vi "DevTests_TestEvent.vi"() -> ()   [LabVIEW 2024]
uses:
  SDL3/Video/WindowFlags--ring.ctl
  SDL3/Pixels/PixelFormat--enum.ctl
  SDL3/Render/TextureAccess-enum.ctl
  SDL3/Error/GetError-UiThread.vi
  SDL3/Pixels/PixelFormatEnumToU32.vi
  <vilib>/Utility/error.llb/Error Cluster From Error Code.vi
  SDL3/Render/Render.lvlib
  SDL3/Init/Init.lvlib
  SDL3/Video/Video.lvlib
  SDL3/Pixels/Pixels.lvlib
  SDL3/Events/Events.lvlib
panel:
  in  "stop":bool
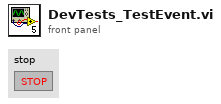
[diagram p1: front panel]
types:
  T1 = typedef "SDL3.lvlib/Render.lvlib/TextureAccess-enum.ctl" = enum32{"SDL_TEXTUREACCESS_STATIC", "SDL_TEXTUREACCESS_STREAMING", "SDL_TEXTUREACCESS_TARGET"}
  T2 = typedef "SDL3.lvlib/Pixels.lvlib/PixelFormat--enum.ctl" = enum32{"SDL_PIXELFORMAT_UNKNOWN", "SDL_PIXELFORMAT_INDEX1LSB", "SDL_PIXELFORMAT_INDEX1MSB", "SDL_PIXELFORMAT_INDEX2LSB", "SDL_PIXELFORMAT_INDEX2MSB", "SDL_PIXELFORMAT_INDEX4LSB", "SDL_PIXELFORMAT_INDEX4MSB", "SDL_PIXELFORMAT_INDEX8", "SDL_PIXELFORMAT_RGB332", "SDL_PIXELFORMAT_XRGB4444", "SDL_PIXELFORMAT_XBGR4444", "SDL_PIXELFORMAT_XRGB1555", "SDL_PIXELFORMAT_XBGR1555", "SDL_PIXELFORMAT_ARGB4444", "SDL_PIXELFORMAT_RGBA4444", "SDL_PIXELFORMAT_ABGR4444", "SDL_PIXELFORMAT_BGRA4444", "SDL_PIXELFORMAT_ARGB1555", "SDL_PIXELFORMAT_RGBA5551", "SDL_PIXELFORMAT_ABGR1555", "SDL_PIXELFORMAT_BGRA5551", "SDL_PIXELFORMAT_RGB565", "SDL_PIXELFORMAT_BGR565", "SDL_PIXELFORMAT_RGB24", "SDL_PIXELFORMAT_BGR24", "SDL_PIXELFORMAT_XRGB8888", "SDL_PIXELFORMAT_RGBX8888", "SDL_PIXELFORMAT_XBGR8888", "SDL_PIXELFORMAT_BGRX8888", "SDL_PIXELFORMAT_ARGB8888", "SDL_PIXELFORMAT_RGBA8888", "SDL_PIXELFORMAT_ABGR8888", "SDL_PIXELFORMAT_BGRA8888", "SDL_PIXELFORMAT_XRGB2101010", "SDL_PIXELFORMAT_XBGR2101010", "SDL_PIXELFORMAT_ARGB2101010", "SDL_PIXELFORMAT_ABGR2101010", "SDL_PIXELFORMAT_RGB48", "SDL_PIXELFORMAT_BGR48", "SDL_PIXELFORMAT_RGBA64", "SDL_PIXELFORMAT_ARGB64", "SDL_PIXELFORMAT_BGRA64", "SDL_PIXELFORMAT_ABGR64", "SDL_PIXELFORMAT_RGB48_FLOAT", "SDL_PIXELFORMAT_BGR48_FLOAT", "SDL_PIXELFORMAT_RGBA64_FLOAT", "SDL_PIXELFORMAT_ARGB64_FLOAT", "SDL_PIXELFORMAT_BGRA64_FLOAT", "SDL_PIXELFORMAT_ABGR64_FLOAT", "SDL_PIXELFORMAT_RGB96_FLOAT", "SDL_PIXELFORMAT_BGR96_FLOAT", "SDL_PIXELFORMAT_RGBA128_FLOAT", "SDL_PIXELFORMAT_ARGB128_FLOAT", "SDL_PIXELFORMAT_BGRA128_FLOAT", "SDL_PIXELFORMAT_ABGR128_FLOAT", "SDL_PIXELFORMAT_YV12", "SDL_PIXELFORMAT_IYUV", "SDL_PIXELFORMAT_YUY2", "SDL_PIXELFORMAT_UYVY", "SDL_PIXELFORMAT_YVYU", "SDL_PIXELFORMAT_NV12", "SDL_PIXELFORMAT_NV21", "SDL_PIXELFORMAT_P010", "SDL_PIXELFORMAT_EXTERNAL_OES"}
  T3 = typedef "SDL3.lvlib/Video.lvlib/WindowFlags--ring.ctl" = u64
  T4 = typedef "SDL3.lvlib/Events.lvlib/EventType--enum.ctl" = enum16{"LV_NONE", "LV_UNSUPPORTED", "SDL_EVENT_QUIT", "SDL_EVENT_LOCALE_CHANGED", "SDL_EVENT_SYSTEM_THEME_CHANGED", "SDL_EVENT_DISPLAY_ORIENTATION", "SDL_EVENT_DISPLAY_ADDED", "SDL_EVENT_DISPLAY_REMOVED", "SDL_EVENT_DISPLAY_MOVED", "SDL_EVENT_DISPLAY_DESKTOP_MODE_CHANGED", "SDL_EVENT_DISPLAY_CURRENT_MODE_CHANGED", "SDL_EVENT_DISPLAY_CONTENT_SCALE_CHANGED", "SDL_EVENT_WINDOW_SHOWN", "SDL_EVENT_WINDOW_HIDDEN", "SDL_EVENT_WINDOW_EXPOSED", "SDL_EVENT_WINDOW_MOVED", "SDL_EVENT_WINDOW_RESIZED", "SDL_EVENT_WINDOW_PIXEL_SIZE_CHANGED", "SDL_EVENT_WINDOW_METAL_VIEW_RESIZED", "SDL_EVENT_WINDOW_MINIMIZED", "SDL_EVENT_WINDOW_MAXIMIZED", "SDL_EVENT_WINDOW_RESTORED", "SDL_EVENT_WINDOW_MOUSE_ENTER", "SDL_EVENT_WINDOW_MOUSE_LEAVE", "SDL_EVENT_WINDOW_FOCUS_GAINED", "SDL_EVENT_WINDOW_FOCUS_LOST", "SDL_EVENT_WINDOW_CLOSE_REQUESTED", "SDL_EVENT_WINDOW_HIT_TEST", "SDL_EVENT_WINDOW_ICCPROF_CHANGED", "SDL_EVENT_WINDOW_DISPLAY_CHANGED", "SDL_EVENT_WINDOW_DISPLAY_SCALE_CHANGED", "SDL_EVENT_WINDOW_SAFE_AREA_CHANGED", "SDL_EVENT_WINDOW_OCCLUDED", "SDL_EVENT_WINDOW_ENTER_FULLSCREEN", "SDL_EVENT_WINDOW_LEAVE_FULLSCREEN", "SDL_EVENT_WINDOW_DESTROYED", "SDL_EVENT_WINDOW_HDR_STATE_CHANGED", "SDL_EVENT_KEY_DOWN", "SDL_EVENT_KEY_UP", "SDL_EVENT_TEXT_EDITING", "SDL_EVENT_TEXT_INPUT", "SDL_EVENT_KEYMAP_CHANGED", "SDL_EVENT_KEYBOARD_ADDED", "SDL_EVENT_KEYBOARD_REMOVED", "SDL_EVENT_TEXT_EDITING_CANDIDATES", "SDL_EVENT_MOUSE_MOTION", "SDL_EVENT_MOUSE_BUTTON_DOWN", "SDL_EVENT_MOUSE_BUTTON_UP", "SDL_EVENT_MOUSE_WHEEL", "SDL_EVENT_MOUSE_ADDED", "SDL_EVENT_MOUSE_REMOVED", "SDL_EVENT_JOYSTICK_AXIS_MOTION", "SDL_EVENT_JOYSTICK_BALL_MOTION", "SDL_EVENT_JOYSTICK_HAT_MOTION", "SDL_EVENT_JOYSTICK_BUTTON_DOWN", "SDL_EVENT_JOYSTICK_BUTTON_UP", "SDL_EVENT_JOYSTICK_ADDED", "SDL_EVENT_JOYSTICK_REMOVED", "SDL_EVENT_JOYSTICK_BATTERY_UPDATED", "SDL_EVENT_JOYSTICK_UPDATE_COMPLETE", "SDL_EVENT_GAMEPAD_AXIS_MOTION", "SDL_EVENT_GAMEPAD_BUTTON_DOWN", "SDL_EVENT_GAMEPAD_BUTTON_UP", "SDL_EVENT_GAMEPAD_ADDED", "SDL_EVENT_GAMEPAD_REMOVED", "SDL_EVENT_GAMEPAD_REMAPPED", "SDL_EVENT_GAMEPAD_TOUCHPAD_DOWN", "SDL_EVENT_GAMEPAD_TOUCHPAD_MOTION", "SDL_EVENT_GAMEPAD_TOUCHPAD_UP", "SDL_EVENT_GAMEPAD_SENSOR_UPDATE", "SDL_EVENT_GAMEPAD_UPDATE_COMPLETE", "SDL_EVENT_GAMEPAD_STEAM_HANDLE_UPDATED", "SDL_EVENT_FINGER_DOWN", "SDL_EVENT_FINGER_UP", "SDL_EVENT_FINGER_MOTION", "SDL_EVENT_CLIPBOARD_UPDATE", "SDL_EVENT_DROP_FILE", "SDL_EVENT_DROP_TEXT", "SDL_EVENT_DROP_BEGIN", "SDL_EVENT_DROP_COMPLETE", "SDL_EVENT_DROP_POSITION", "SDL_EVENT_AUDIO_DEVICE_ADDED", "SDL_EVENT_AUDIO_DEVICE_REMOVED", "SDL_EVENT_AUDIO_DEVICE_FORMAT_CHANGED", "SDL_EVENT_SENSOR_UPDATE", "SDL_EVENT_PEN_PROXIMITY_IN", "SDL_EVENT_PEN_PROXIMITY_OUT", "SDL_EVENT_PEN_DOWN", "SDL_EVENT_PEN_UP", "SDL_EVENT_PEN_BUTTON_DOWN", "SDL_EVENT_PEN_BUTTON_UP", "SDL_EVENT_PEN_MOTION", "SDL_EVENT_PEN_AXIS", "SDL_EVENT_CAMERA_DEVICE_ADDED", "SDL_EVENT_CAMERA_DEVICE_REMOVED", "SDL_EVENT_CAMERA_DEVICE_APPROVED", "SDL_EVENT_CAMERA_DEVICE_DENIED", "SDL_EVENT_RENDER_TARGETS_RESET", "SDL_EVENT_RENDER_DEVICE_RESET", "SDL_EVENT_POLL_SENTINEL", "SDL_EVENT_USER"}
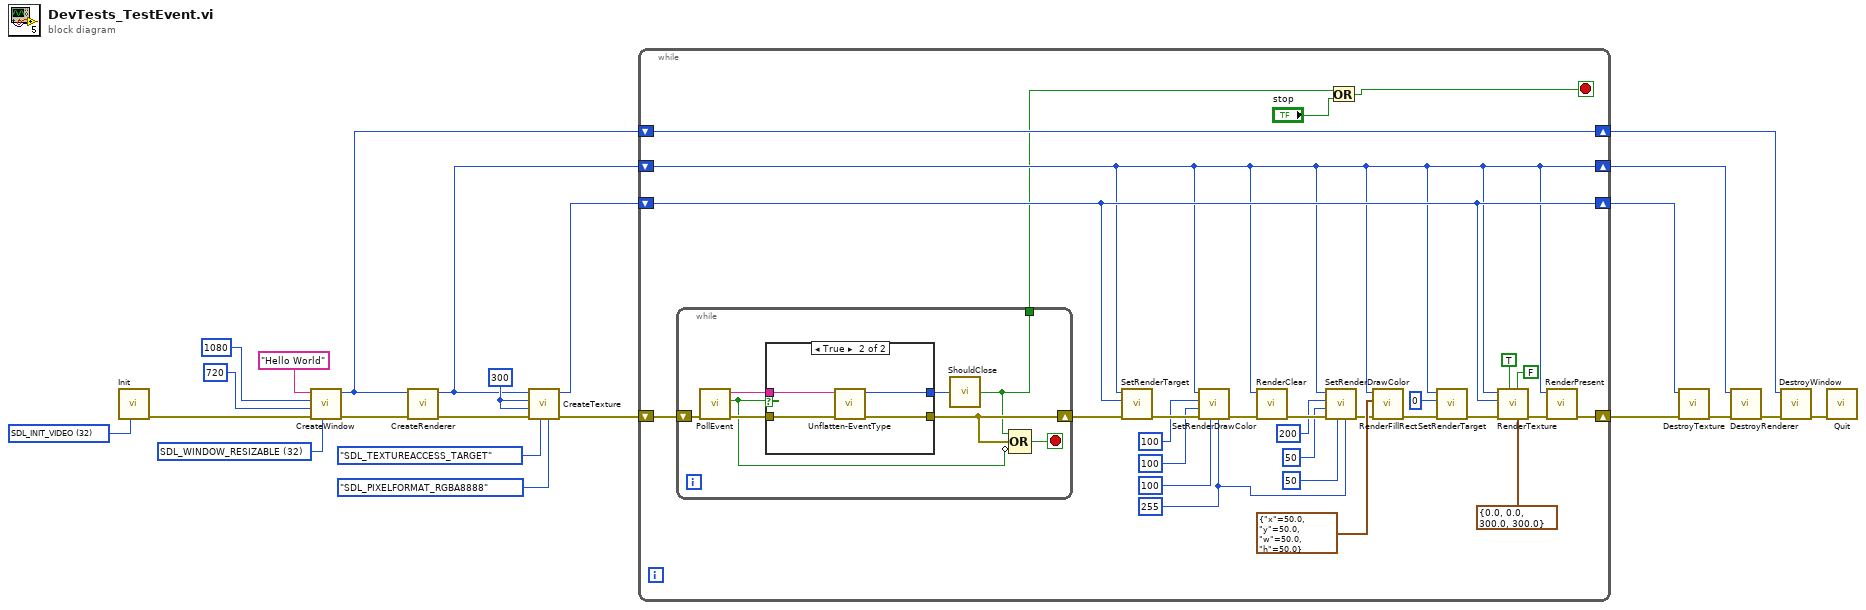
[diagram p0: block diagram]
diagram:
  w14 = 300 ("w")
  w19 = T3 32 items=["0"=0, "SDL_WINDOW_FULLSCREEN"=1, "SDL_WINDOW_OPENGL"=2, "SDL_WINDOW_OCCLUDED"=4, "SDL_WINDOW_HIDDEN"=8, "SDL_WINDOW_BORDERLESS"=16, "SDL_WINDOW_RESIZABLE"=32, "SDL_WINDOW_MINIMIZED"=64, "SDL_WINDOW_MAXIMIZED"=128, "SDL_WINDOW_MOUSE_GRABBED"=256, "SDL_WINDOW_INPUT_FOCUS"=512, "SDL_WINDOW_MOUSE_FOCUS"=1024, "SDL_WINDOW_EXTERNAL"=2048, "SDL_WINDOW_MODAL"=4096, "SDL_WINDOW_HIGH_PIXEL_DENSITY"=8192, "SDL_WINDOW_MOUSE_CAPTURE"=16384, "SDL_WINDOW_MOUSE_RELATIVE_MODE"=32768, "SDL_WINDOW_ALWAYS_ON_TOP"=65536, "SDL_WINDOW_UTILITY"=131072, "SDL_WINDOW_TOOLTIP"=262144, "SDL_WINDOW_POPUP_MENU"=524288, "SDL_WINDOW_KEYBOARD_GRABBED"=1048576, "SDL_WINDOW_VULKAN"=268435456, "SDL_WINDOW_METAL"=536870912, "SDL_WINDOW_TRANSPARENT"=1073741824, "SDL_WINDOW_NOT_FOCUSABLE"=2147483648] ("flags (0)")
  w3 = u32 32 items=["NONE"=0, "SDL_INIT_AUDIO"=16, "SDL_INIT_VIDEO"=32, "SDL_INIT_JOYSTICK"=512, "SDL_INIT_HAPTIC"=4096, "SDL_INIT_GAMEPAD"=8192, "SDL_INIT_EVENTS"=16384, "SDL_INIT_SENSOR"=32768, "SDL_INIT_CAMER"=65536] ("flags")
  n1 = call "Init.vi"("InitFlags"=w3) -> ("error out"=w22:errorcluster)  [unwired: 10 in]
  n2 = call "CreateWindow.vi"("Flags (0)"=w19, "No Error"=w22, "h"=720, "w"=1080, "Title"="Hello World" ("title")) -> ("Error Out"=w18:errorcluster, "Window [SDL_Window *]"=w10:i64)  [unwired: 5 in]
  n3 = call "CreateRenderer.vi"("No Error"=w18, "Window [SDL_Window *]"=w10) -> ("Error Out"=w15:errorcluster, "Renderer [SDL_Renderer *]"=w9:i64)  [unwired: 8 in]
  n4 = call "CreateTexture.vi"("Pixel Format"=PixelFormat--enum."SDL_PIXELFORMAT_RGBA8888" ("pixel_format"), "Texture Access"=TextureAccess-enum."SDL_TEXTUREACCESS_TARGET" ("texture_access"), "No Error"=w15, "h"=w14, "w"=w14, "Renderer [SDL_Renderer *]"=w9) -> ("error out"=w4:errorcluster, "Texture [SDL_Texture *]"=w8:i64)  [unwired: 4 in]
  n5 = while {
    shift-right: [w38] -> w5
    shift-left: w8 -> [w38]
    shift-right: [w33] -> w6
    shift-left: w9 -> [w33]
    shift-right: [w50] -> w7
    shift-left: w10 -> [w50]
    shift-right: [w39] -> w17
    shift-left: w4 -> [w23]
    stop <- w26 stop-if-true
    w29 = u8 255 ("a")
    n6 = while {
      shift-right: [w53] -> w27
      shift-left: w23 -> [w58]
      tunnel: [w51] -> w24
      stop <- w57 stop-if-true
      n7 = call "PollEvent.vi"("No Error"=w58) -> ("error out"=w56:errorcluster, "Event Occured?"=w54:bool, "Event Binary Data"=w55:string)  [unwired: 8 in]
      n8 = case shown="True" w54 {
        tunnel: w56 -> [w59 w63]
        tunnel: w55 -> [_ w62]
        tunnel: [w59 w61] -> w53
        tunnel: [_ w60] -> w52
        frame False {
        }
        frame True {
          n9 = call "Unflatten-EventType.vi"("error in (no error)"=w63, "Event Binary Data In"=w62) -> ("error out"=w61:errorcluster, "EventType"=w60:T4)  [unwired: 8 in]
        }
      }
      n10 = call "ShouldClose.vi"("EventType"=w52) -> ("Close?"=w51:bool)
      n11 = Compound Arithmetic op=OR(w51, w53, invert w54) -> (w57:bool)
    }
    n12 = call "SetRenderTarget.vi"("No Error"=w27, "Texture [SDL_Texture *]"=w38, "Renderer [SDL_Renderer *]"=w33) -> ("error out"=w47:errorcluster)  [unwired: 8 in]
    n13 = call "SetRenderDrawColor.vi"("a"=w29, "b"=u8 100, "No Error"=w47, "g"=u8 100, "r"=u8 100, "Renderer [SDL_Renderer *]"=w33) -> ("error out"=w45:errorcluster)  [unwired: 5 in]
    n14 = call "RenderClear.vi"("No Error"=w45, "Renderer [SDL_Renderer *]"=w33) -> ("error out"=w46:errorcluster)  [unwired: 9 in]
    n15 = call "SetRenderDrawColor.vi"("a"=w29, "b"=u8 50, "No Error"=w46, "g"=u8 50, "r"=u8 200, "Renderer [SDL_Renderer *]"=w33) -> ("error out"=w34:errorcluster)  [unwired: 5 in]
    n16 = Or(x=w24, y="stop") -> (x .or. y?=w26:bool)
    n17 = call "RenderFillRect.vi"("No Error"=w34, "Rect"=cluster{"x":sgl, "y":sgl, "w":sgl, "h":sgl} {"x"=50.0, "y"=50.0, "w"=50.0, "h"=50.0} ("rect"), "Renderer [SDL_Renderer *]"=w33) -> ("error out"=w28:errorcluster)  [unwired: 8 in]
    n18 = call "SetRenderTarget.vi"("No Error"=w28, "Texture [SDL_Texture *]"=i64 0 ("texture [SDL_Texture *]"), "Renderer [SDL_Renderer *]"=w33) -> ("error out"=w48:errorcluster)  [unwired: 8 in]
    n19 = call "RenderTexture.vi"("Dstrect"=cluster{"x":sgl, "y":sgl, "w":sgl, "h":sgl} {"x"=0.0, "y"=0.0, "w"=300.0, "h"=300.0} ("dstrect"), "Entire Rendering Target (F)"=FALSE, "Entire Texture (F)"=TRUE, "No Error"=w48, "Texture [SDL_Texture *]"=w38, "Renderer [SDL_Renderer *]"=w33) -> ("error out"=w49:errorcluster)  [unwired: 5 in]
    n20 = call "RenderPresent.vi"("No Error"=w49, "Renderer [SDL_Renderer *]"=w33) -> ("error out"=w39:errorcluster)  [unwired: 9 in]
  }
  n21 = call "DestroyTexture.vi"("No Error"=w17, "Texture [SDL_Texture *]"=w5) -> ("error out"=w11:errorcluster)  [unwired: 9 in]
  n22 = call "DestroyRenderer.vi"("No Error"=w11, "Rrenderer [SDL_Renderer *]"=w6) -> ("error out"=w16:errorcluster)  [unwired: 9 in]
  n23 = call "DestroyWindow.vi"("No Error"=w16, "Window [SDL_Window*]"=w7) -> ("Error Out"=w21:errorcluster)  [unwired: 9 in]
  n24 = call "Quit.vi"("No Error"=w21) -> ()  [unwired: 10 in, 1 out]
